vi "Edge Tetector.vi"(8 "error in (no error)":errorcluster, 11 "Refnum in":T1) -> (0 "error out":errorcluster, 3 "Refnum out":T1)   [LabVIEW 2015]
uses:
  <vilib>/vision/Image Controls.llb/IMAQ Image.ctl
  <vilib>/vision/NI_Vision_Development_Module.lvlib
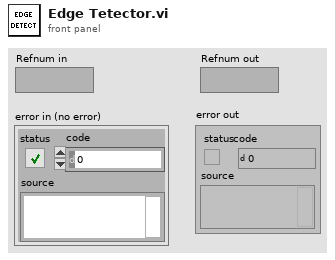
[diagram p1: front panel]
types:
  T1 = typedef "IMAQ Image.ctl" = refnum<image>
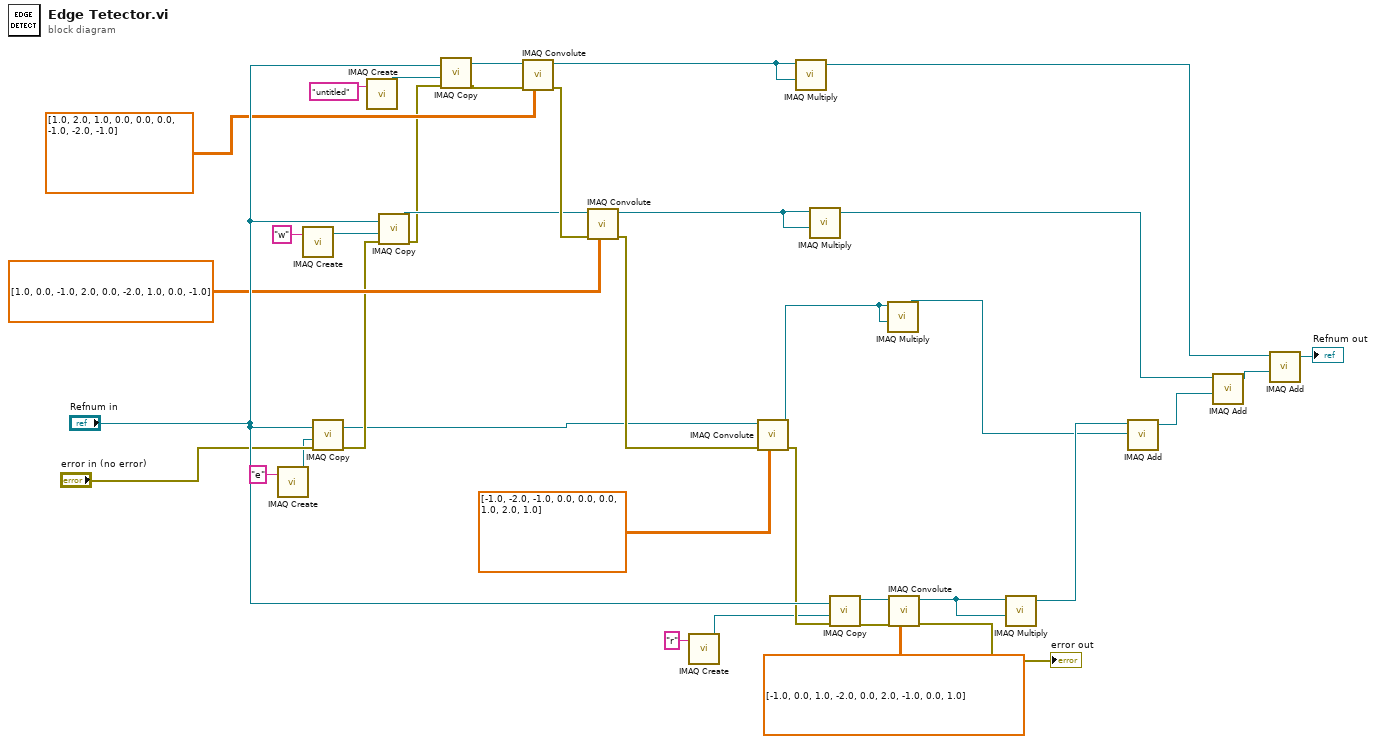
[diagram p0: block diagram]
diagram:
  n1 = call "IMAQ Create"("Image Name"="e") -> ("New Image"=w3:T1)  [unwired: 4 in, 1 out]
  n2 = call "IMAQ Create"("Image Name"="w") -> ("New Image"=w10:T1)  [unwired: 4 in, 1 out]
  n3 = call "IMAQ Copy"("error in (no error)"="error in (no error)", "Image Dst"=w3, "Image Src"="Refnum in") -> ("error out"=w12:errorcluster, "Image Dst Out"=w5:T1)  [unwired: 3 in]
  n4 = call "IMAQ Create"("Image Name"="untitled") -> ("New Image"=w11:T1)  [unwired: 4 in, 1 out]
  n5 = call "IMAQ Copy"("error in (no error)"=w12, "Image Dst"=w10, "Image Src"="Refnum in") -> ("error out"=w13:errorcluster, "Image Dst Out"=w15:T1)  [unwired: 3 in]
  n6 = call "IMAQ Copy"("error in (no error)"=w13, "Image Dst"=w11, "Image Src"="Refnum in") -> ("error out"=w19:errorcluster, "Image Dst Out"=w16:T1)  [unwired: 3 in]
  n7 = call "IMAQ Convolute"("Kernel"=sgl[][] [[1.0, 2.0, 1.0], [0.0, 0.0, 0.0], [-1.0, -2.0, -1.0]] ("transposed array"), "error in (no error)"=w19, "Image Src"=w16) -> ("error out"=w20:errorcluster, "Image Dst Out"=w23:T1)  [unwired: 4 in, 3 out]
  n8 = call "IMAQ Convolute"("Kernel"=sgl[][] [[1.0, 0.0, -1.0], [2.0, 0.0, -2.0], [1.0, 0.0, -1.0]], "error in (no error)"=w20, "Image Src"=w15) -> ("error out"=w21:errorcluster, "Image Dst Out"=w35:T1)  [unwired: 4 in, 3 out]
  n9 = call "IMAQ Create"("Image Name"="r") -> ("New Image"=w31:T1)  [unwired: 4 in, 1 out]
  n10 = call "IMAQ Convolute"("Kernel"=sgl[][] [[-1.0, -2.0, -1.0], [0.0, 0.0, 0.0], [1.0, 2.0, 1.0]] ("transposed array"), "error in (no error)"=w21, "Image Src"=w5) -> ("error out"=w33:errorcluster, "Image Dst Out"=w26:T1)  [unwired: 4 in, 3 out]
  n11 = call "IMAQ Multiply"("Image Src A"=w23, "Image Src B"=w23) -> ("Image Dst Out"=w24:T1)  [unwired: 5 in, 1 out]
  n12 = call "IMAQ Multiply"("Image Src A"=w35, "Image Src B"=w35) -> ("Image Dst Out"=w25:T1)  [unwired: 5 in, 1 out]
  n13 = call "IMAQ Copy"("error in (no error)"=w33, "Image Dst"=w31, "Image Src"="Refnum in") -> ("error out"=w34:errorcluster, "Image Dst Out"=w32:T1)  [unwired: 3 in]
  n14 = call "IMAQ Multiply"("Image Src A"=w26, "Image Src B"=w26) -> ("Image Dst Out"=w27:T1)  [unwired: 5 in, 1 out]
  n15 = call "IMAQ Convolute"("Kernel"=sgl[][] [[-1.0, 0.0, 1.0], [-2.0, 0.0, 2.0], [-1.0, 0.0, 1.0]], "error in (no error)"=w34, "Image Src"=w32) -> ("error out"=→"error out":errorcluster, "Image Dst Out"=w28:T1)  [unwired: 4 in, 3 out]
  n16 = call "IMAQ Multiply"("Image Src A"=w28, "Image Src B"=w28) -> ("Image Dst Out"=w29:T1)  [unwired: 5 in, 1 out]
  n17 = call "IMAQ Add"("Image Src A"=w29, "Image Src B"=w27) -> ("Image Dst Out"=w18:T1)  [unwired: 5 in, 1 out]
  n18 = call "IMAQ Add"("Image Src A"=w25, "Image Src B"=w18) -> ("Image Dst Out"=w17:T1)  [unwired: 5 in, 1 out]
  n19 = call "IMAQ Add"("Image Src A"=w24, "Image Src B"=w17) -> ("Image Dst Out"=→"Refnum out":T1)  [unwired: 5 in, 1 out]
